vi "Open.vi"(0 "DeviceNumber":i32) -> (1 "DeviceHandle":i32, 2 "Error":bool)   [LabVIEW 2012]
uses:
  MPS-060602.dll
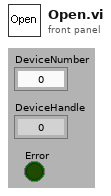
[diagram p1: front panel]
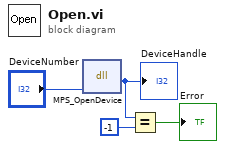
[diagram p0: block diagram]
diagram:
  n1 = dll-call lib="PTH1Yabs CDocuments and Settings\nAdministrator桌面性能\tdriver VIMPS-060602.dll" fn="MPS_OpenDevice"("DeviceNumber"="DeviceNumber") -> (w3:i32)  [unwired: 4 in, 2 out]
  "DeviceHandle" <- w3
  n2 = Equal?(x=w3, y=-1) -> (x = y?=→"Error":bool)
